vi "STORE_LINEBACK.vi"(9 "CURRENT_YEAR_DATA":string, 10 "ECODE 2":string, 11 "connection reference":T1) -> ()   [LabVIEW 2015]
uses:
  <vilib>/addons/database/Connection.llb/Conn ObjectReference.ctl
  Controls/ITEM_INFORMATION_CLUSTER.ctl
  Controls/Print_Data.ctl
  <vilib>/Instr/_visa.llb/VISA Configure Serial Port (Instr).vi
  <vilib>/addons/database/_DB Variant To Data/Database Variant To Data.xnode
  <vilib>/addons/database/NI_Database_API.lvlib
  <vilib>/addons/database/Connection.llb/DB Tools Open Connec (String).vi
panel:
  in  "Print Button":bool
  in  "BUTTON_ADD":bool
  in  "AUTO PRINT":bool
  in  "Lot Maker":string
  out "Invoice Date":timestamp format="%<%d/%m/%Y>T"
  in  "Location":string
  in  "Scale":refnum<visa-resource-name>
  in  "Tare (g)":dbl
  in  "Weight":dbl
  in  "Sample":dbl caption="Sample (Unit/g)"
  in  "Maker Code":string
  in  "Invoice No.":string
  in  "BUTTON_EXIT":bool
  in  "BUTTON_INPUT":bool
  in  "Unit 2":string
  in  "Quantity":dbl
  in  "Item Code":string
  in  "QR Code (F3)":string
  in  "Maker":string
  in  "Part Name":string
  in  "Product":string
  out "ECODE":string
  out "Lineback Date":timestamp format="%<%d/%m/%Y>T"
  in  "Line No.(F1)":string
  # "INPUT  FROM LINE"
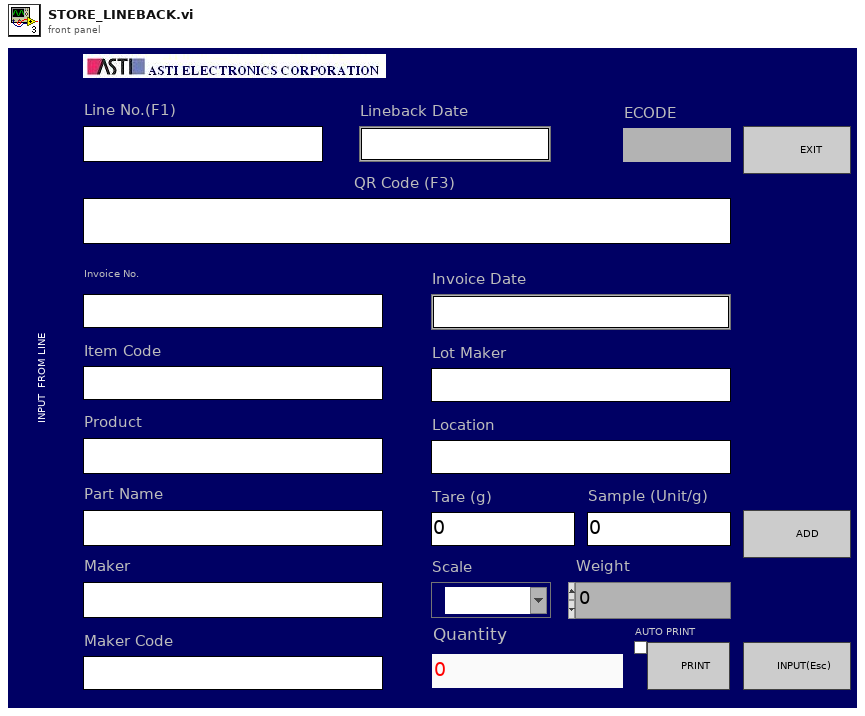
[diagram p1: front panel]
types:
  T1 = typedef "NI_Database_API.lvlib/Conn ObjectReference.ctl" = refnum<k1>
  T2 = cluster{"INVOICE_DATE":timestamp, "LOT_MAKER":string, "INVOICE_NO":string}[]
  T3 = typedef "ITEM_INFORMATION_CLUSTER.ctl" = cluster{"PRODUCT":string, "ITEM_CODE":string, "PART_NAME":string, "MAKER":string, "PART_NO":string, "LOT_SIZE":dbl, "UNIT":string, "LENGTH-OFFSET":string, "BARCODE":string, "PROCESS":string, "INVENTORY_LOCAL":string, "TARE":dbl, "SAMPLE":dbl}
  T4 = cluster{"PRODUCT":string, "ITEM CODE":string, "PART NAME":string, "MAKER":string, "PART NO":string, "LOT SIZE":dbl, "UNIT":string, "LENGTH-OFFSET":string, "BARCODE":string, "PROCESS":string, "INVENTORY LOCAL":string, "TARE":dbl, "SAMPLE":dbl}
  T5 = cluster{"ITEM_CODE":string, "INVOICE_NO":string, "INVOICE_DATE":timestamp, "LOT_MAKER":string, "QUANTITY":dbl, "INVOICE_ECODE":string, "INPUT_NO":string, "INPUT_DATE":timestamp, "INPUT_ECODE":string, "LINEBACK_NO":string, "LINEBACK_DATE":timestamp, "LINEBACK_ECODE":string, "OUTPUT_NO":string, "OUTPUT_DATE":timestamp, "OUTPUT_ECODE":string, "DESTINATION":string}
  T6 = typedef "Print_Data.ctl" = cluster{"QR_code Text":string, "Lot Maker":string, "Item Code (F3)":string, "date/time string":string, "Invoice No.":string, "Maker":string, "Part No.(F2) ":string, "Location":string, "Product":string, "Qty":string, "ECODE":string}
  T7 = cluster{"INVOICE_DATE":timestamp, "LOT_MAKER":string, "INVOICE_NO":string}
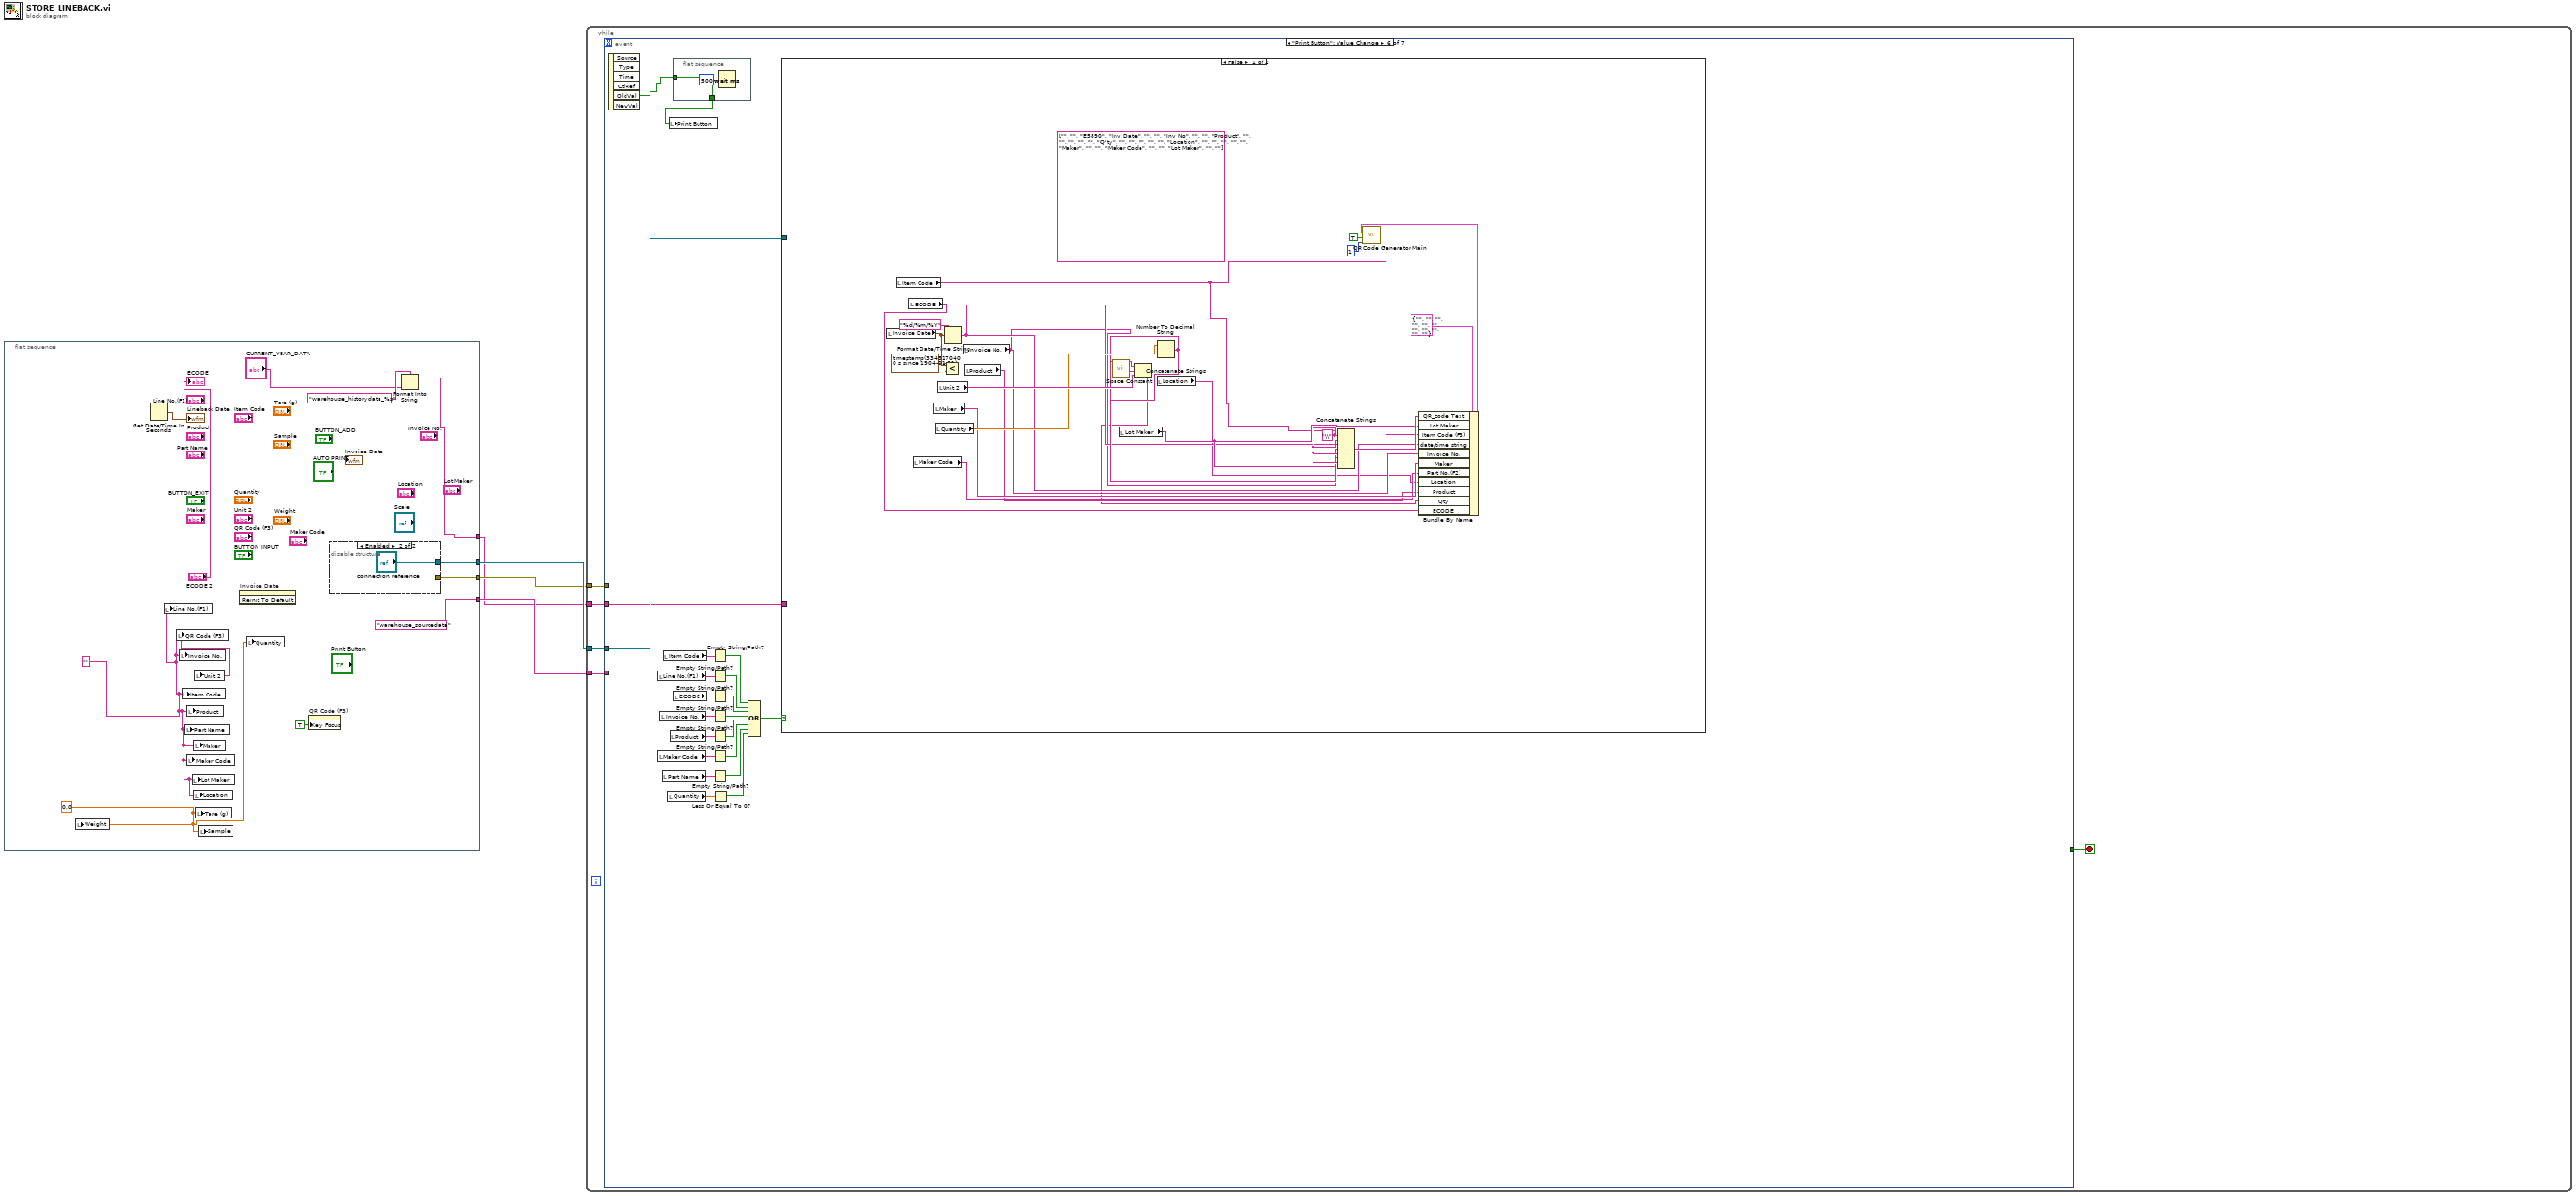
[diagram p0: block diagram]
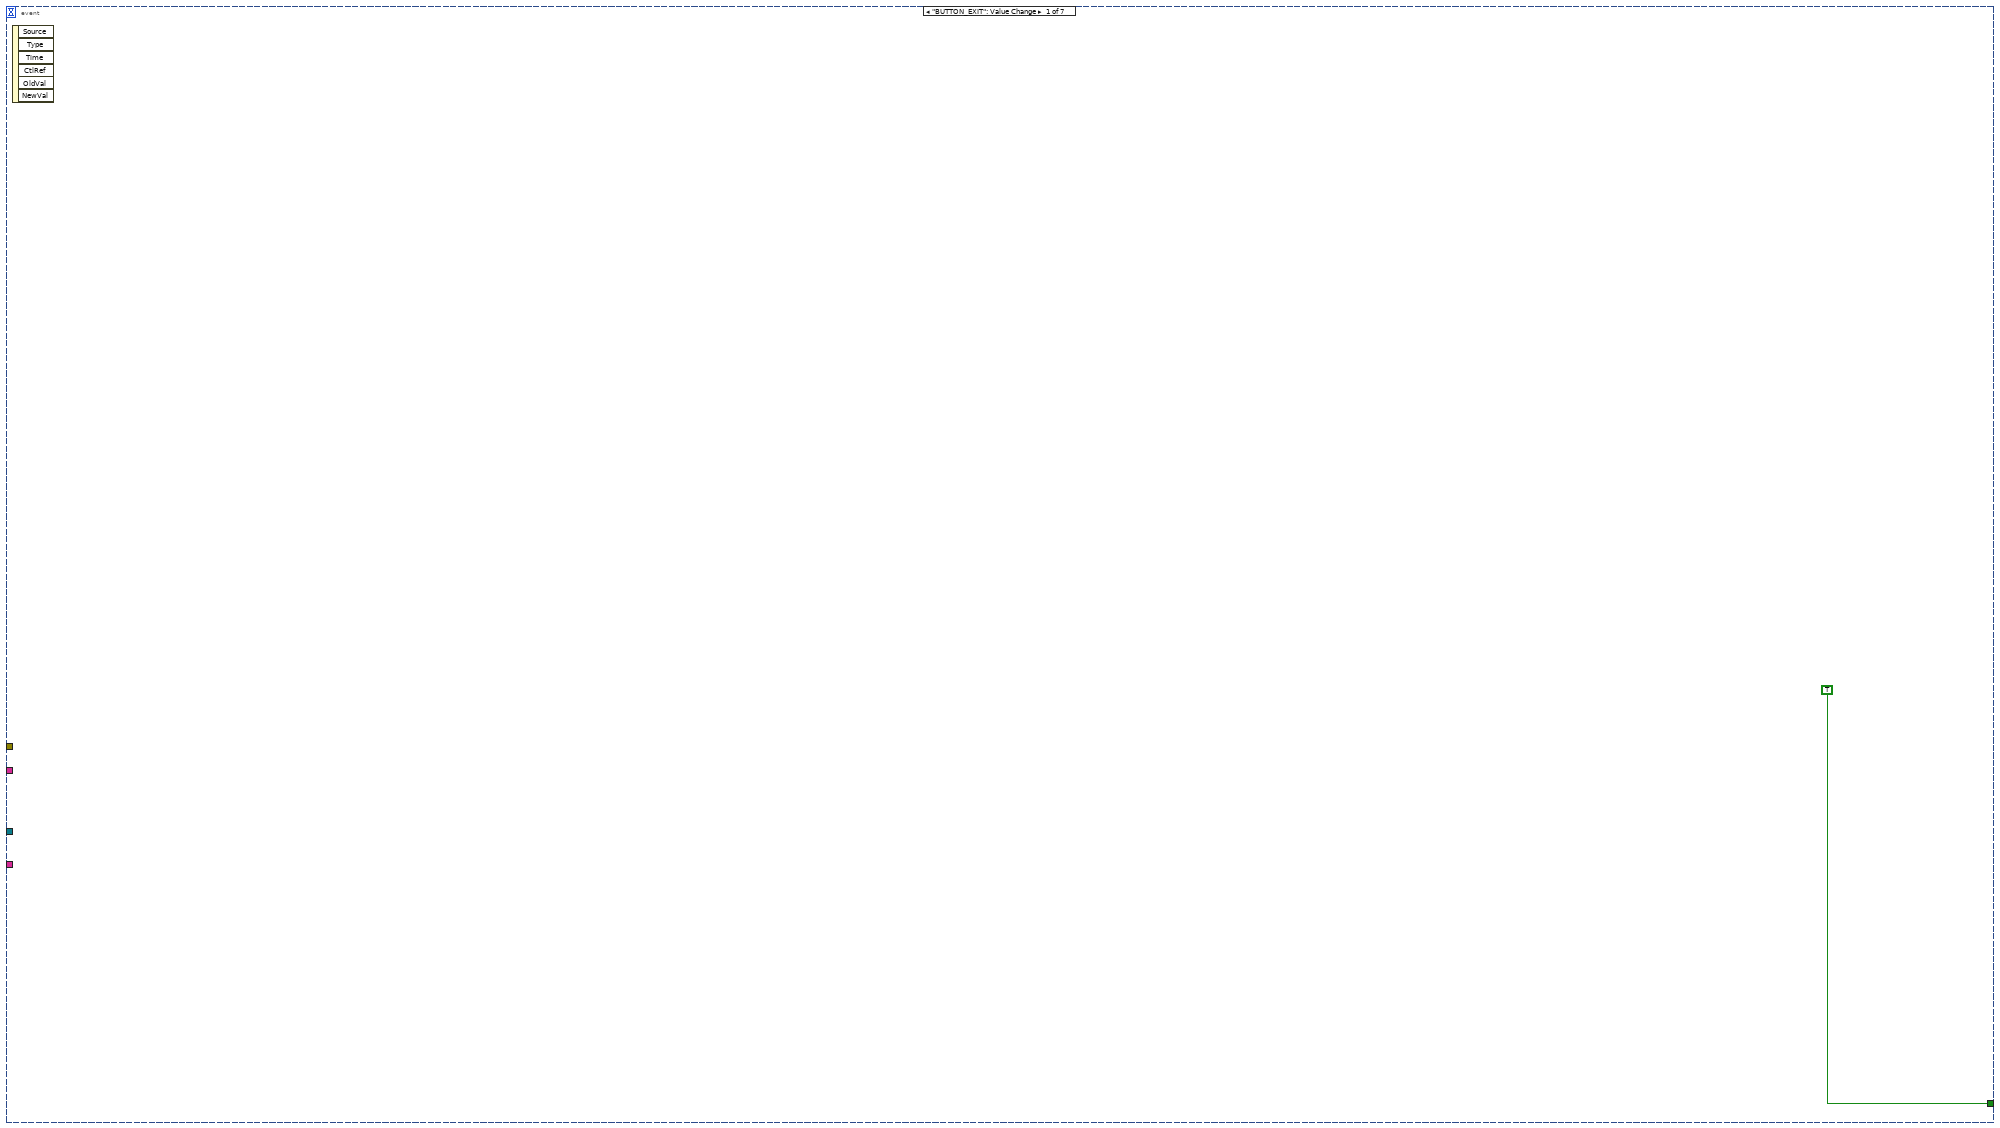
[diagram p2: hidden frame]
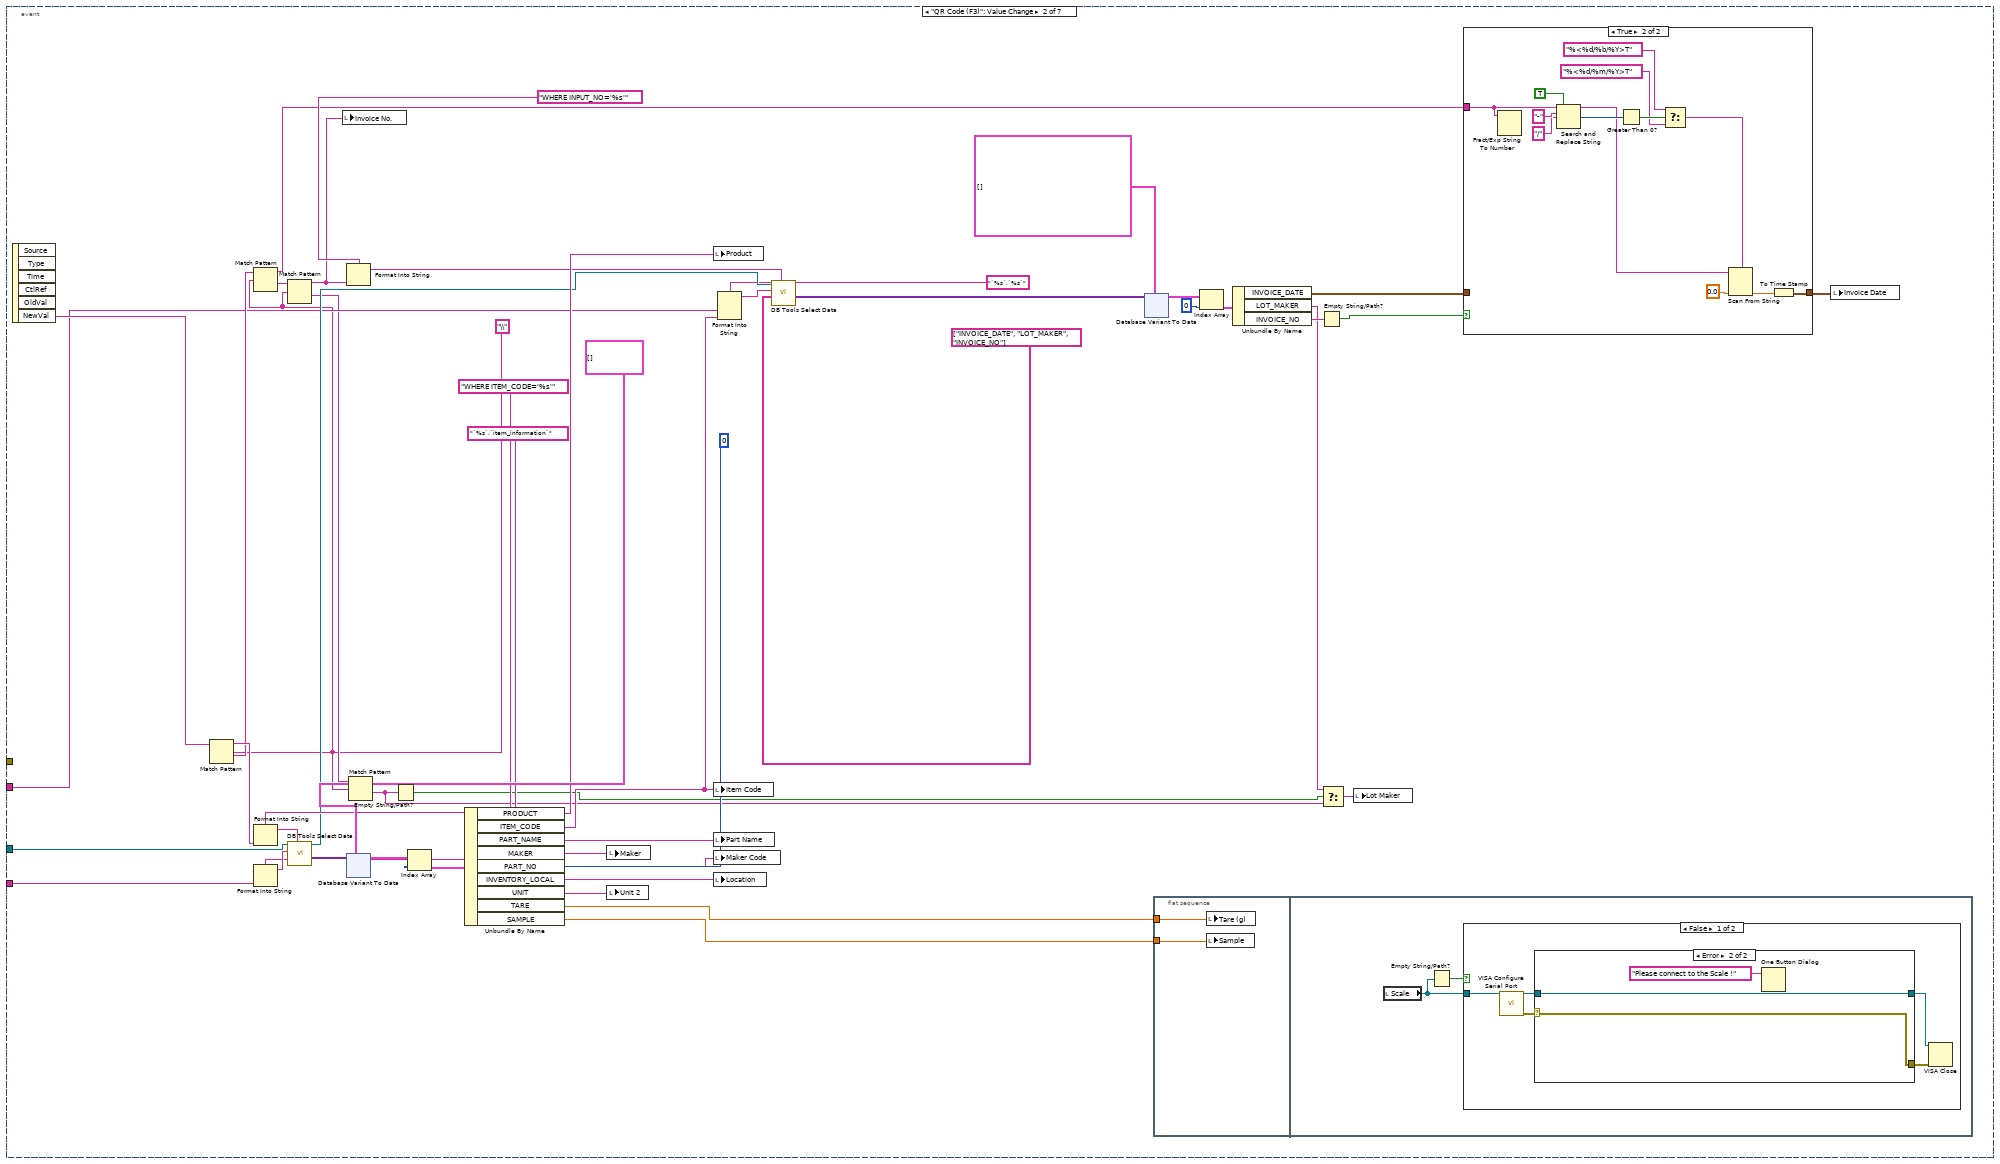
[diagram p3: hidden frame]
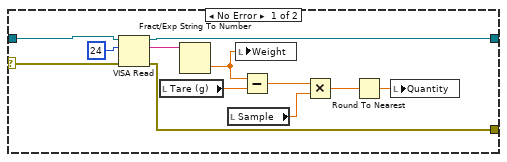
[diagram p5: hidden frame]
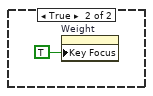
[diagram p6: hidden frame]
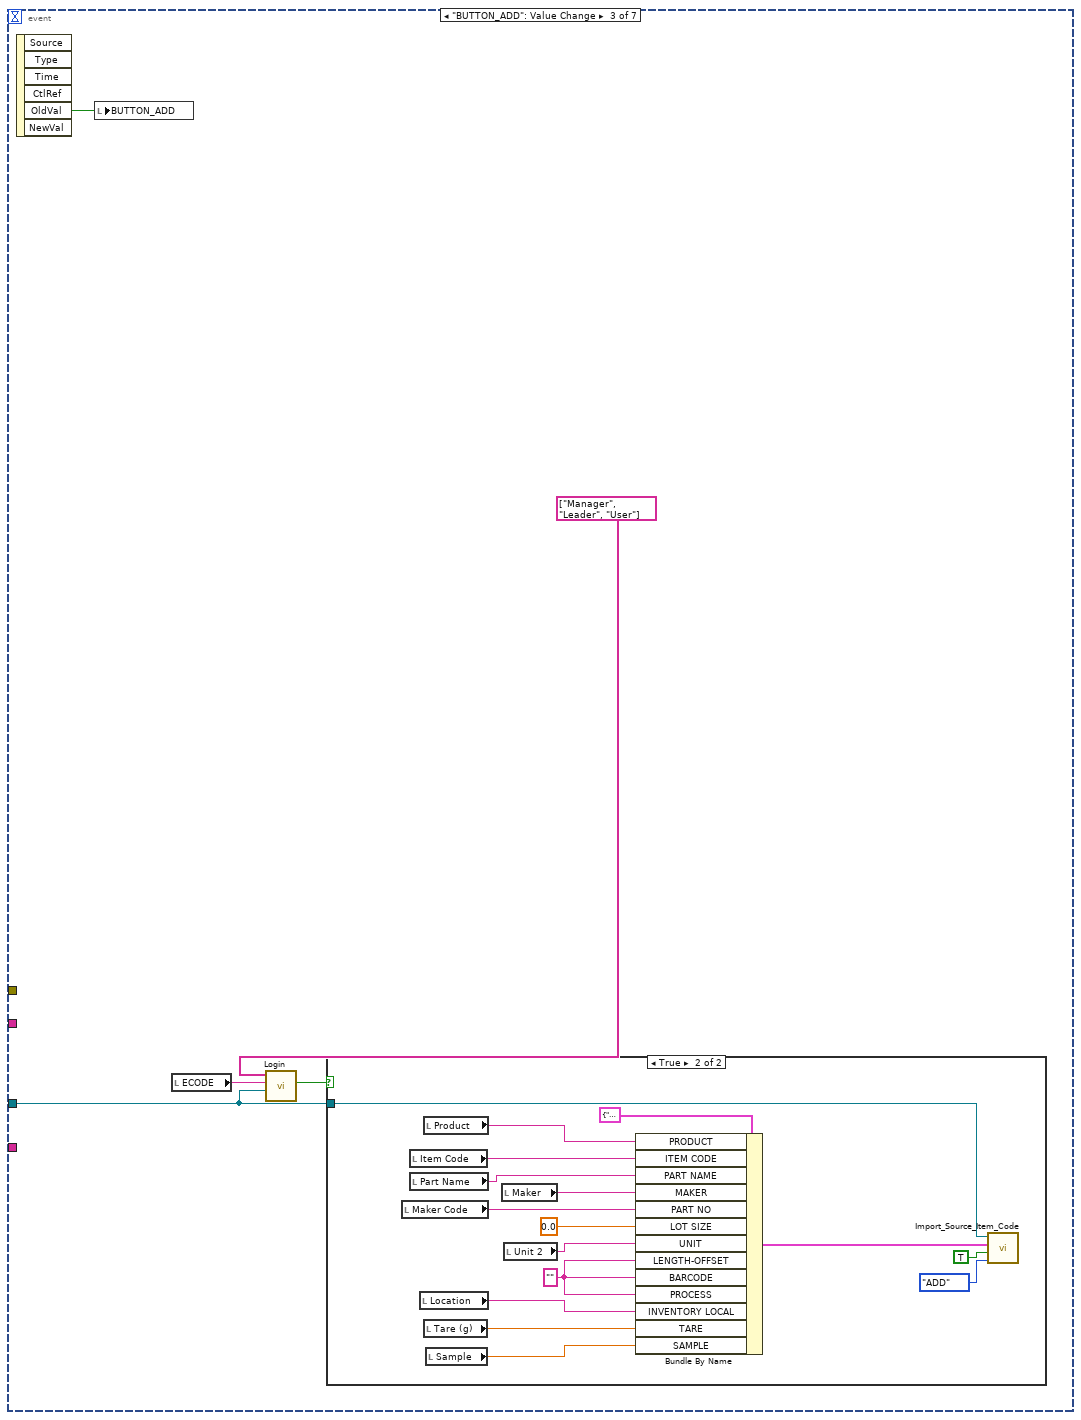
[diagram p7: hidden frame]
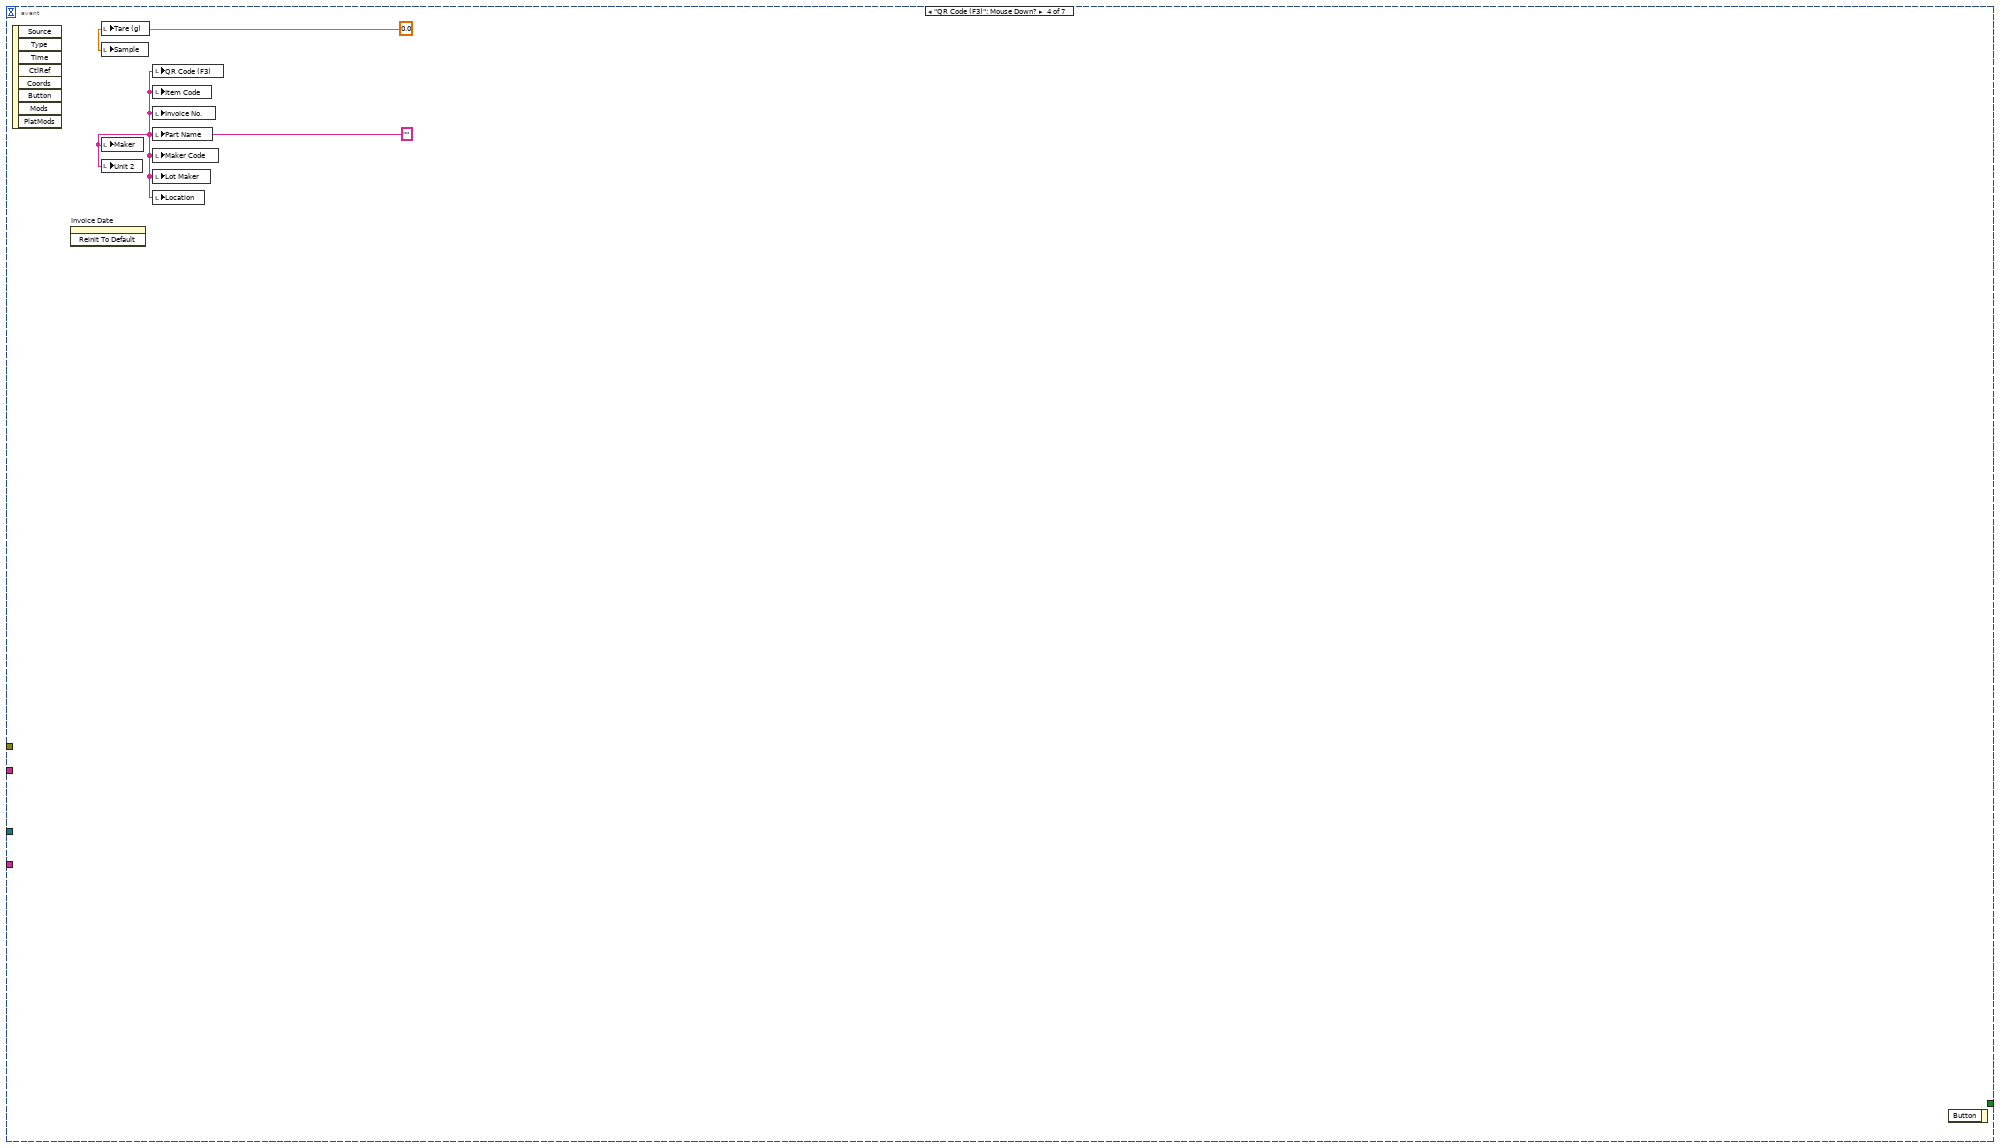
[diagram p9: hidden frame]
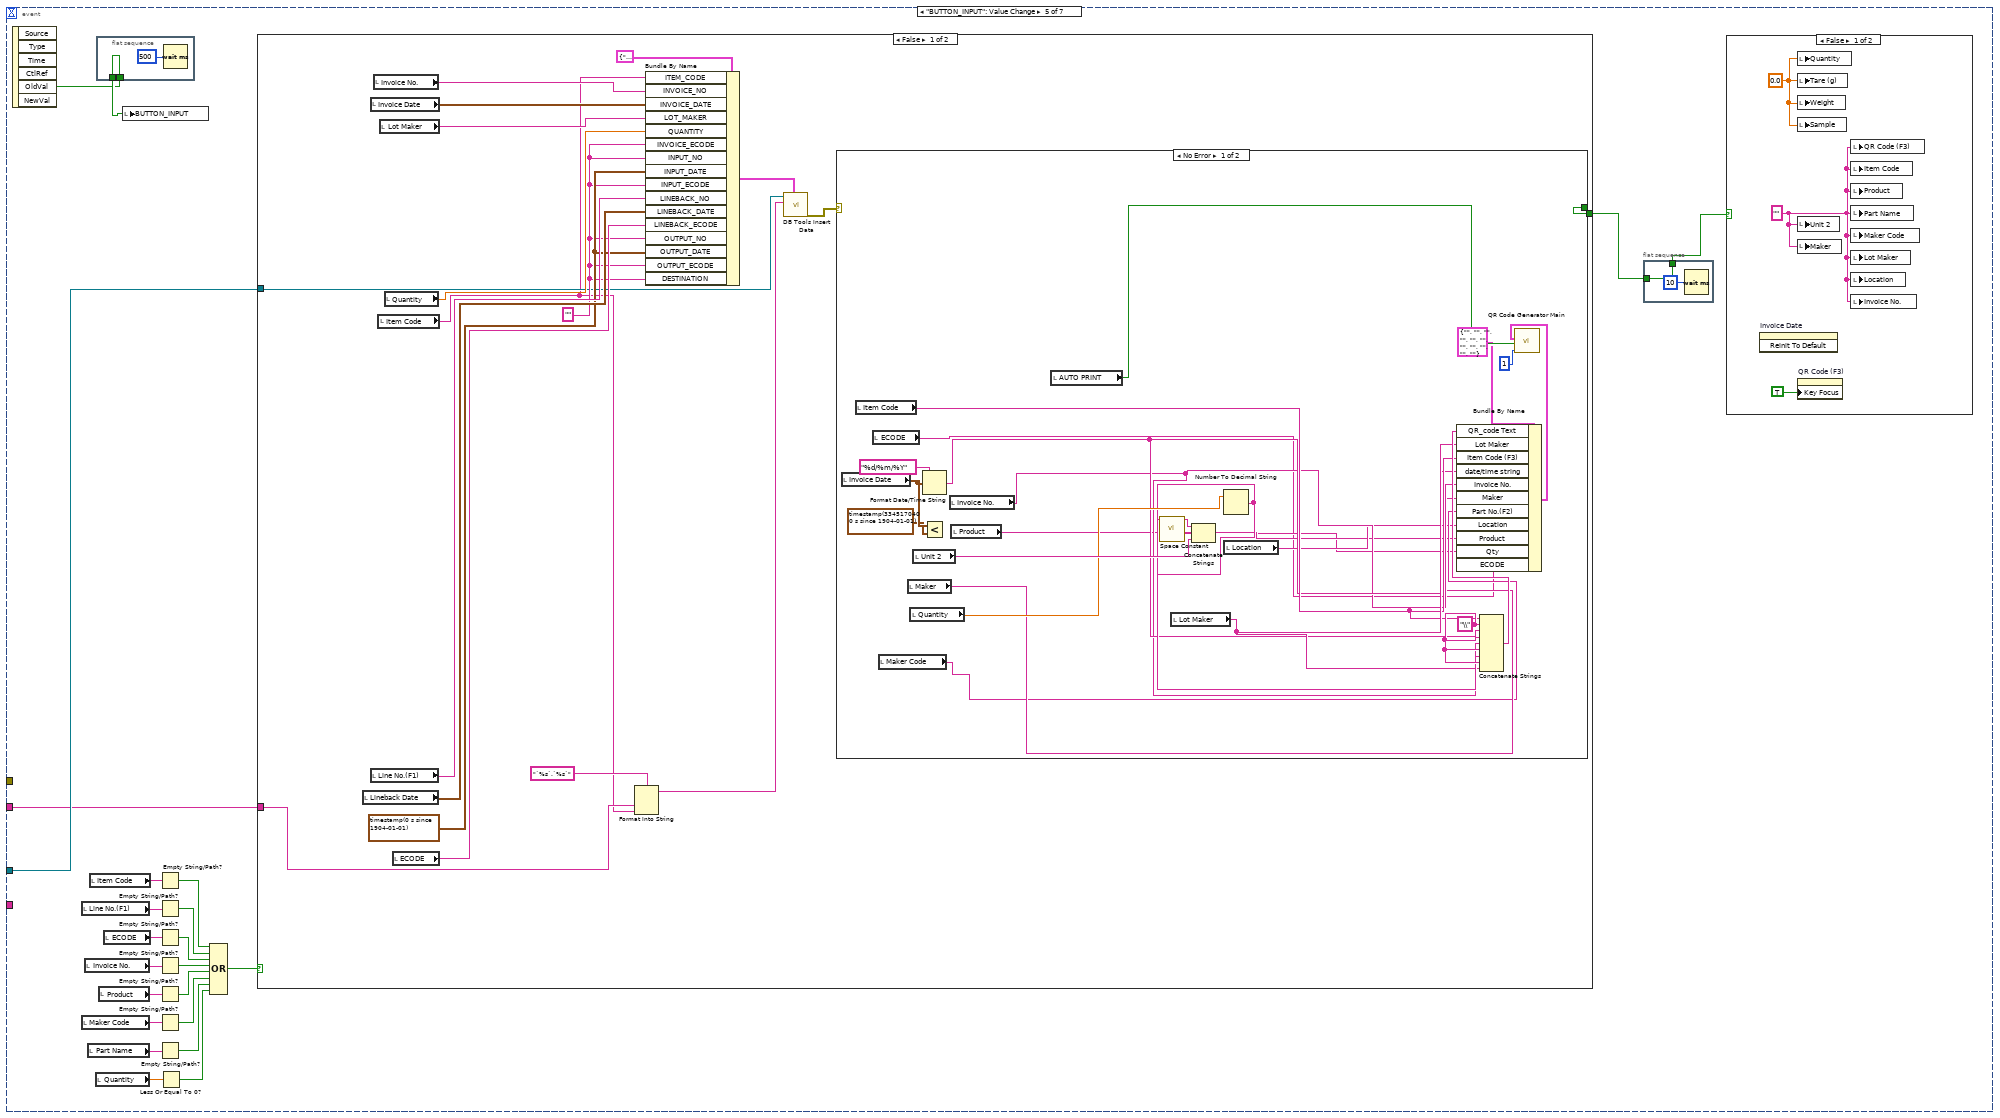
[diagram p10: hidden frame]
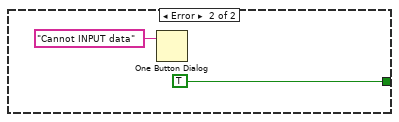
[diagram p12: hidden frame]
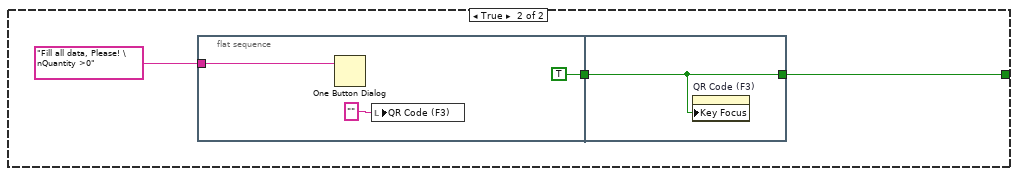
[diagram p13: hidden frame]
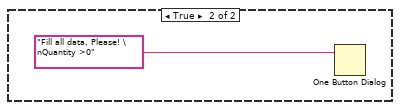
[diagram p14: hidden frame]
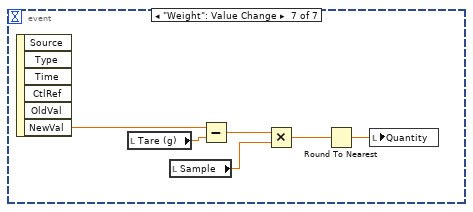
[diagram p15: hidden frame]
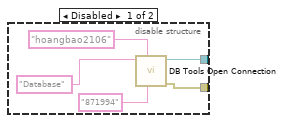
[diagram p16: hidden frame]
diagram:
  n1 = flat-sequence {
    tunnel: [w13] -> w1
    tunnel: [w12] -> w4
    tunnel: [w11] -> w3
    tunnel: ["warehouse_sourcedata" ("table")] -> w2
    frame #0 {
      w6 = ""
      w7 = 0.0
      n2 = local write "Weight"(w7) -> ()
      n3 = Get Date/Time In Seconds() -> (seconds since 1Jan1904=→"Lineback Date":timestamp)
      n4 = local write "Line No.(F1)"(w6) -> ()
      n5 = local write "QR Code (F3)"(w6) -> ()
      n6 = local write "Invoice No."(w6) -> ()
      n7 = local write "Item Code"(w6) -> ()
      n8 = local write "Part Name"(w6) -> ()
      n9 = local write "Maker Code"(w6) -> ()
      n10 = local write "Product"(w6) -> ()
      n11 = local write "Lot Maker"(w6) -> ()
      n12 = local write "Maker"(w6) -> ()
      n13 = local write "Location"(w6) -> ()
      n14 = local write "Unit 2"(w6) -> ()
      n15 = local write "Tare (g)"(w7) -> ()
      n16 = local write "Sample"(w7) -> ()
      n17 = invoke on="Invoice Date" class="AbsTime (strict)" method="Reinit To Default"() -> ()  [unwired: 3 in, 3 out]
      n18 = local write "Quantity"(w7) -> ()
      n19 = property on="QR Code (F3)" class="Str"("Key Focus"=TRUE) -> ()  [unwired: 2 in, 2 out]
      n20 = disable-structure shown="Enabled" {
        disable-tunnel: [w17 "connection reference"] -> w12
        disable-tunnel: [w16 _] -> w11
        frame Disabled {
          n21 = call-poly <vilib>:"DB Tools Open Connection.vi"("password"="871994" ("userID"), "userID"="hoangbao2106", "connection information"="Database" ("userID")) -> ("error out"=w16:errorcluster, "connection reference"=w17:T1)  [unwired: 5 in]
        }
        frame Enabled {
        }
      }
      n22 = Format Into String(format string="warehouse_historydata_%s" ("table"), "CURRENT_YEAR_DATA") -> (resulting string=w13:string)  [unwired: 2 in, 1 out]
      "ECODE" <- "ECODE 2"
    }
  }
  n23 = while {
    tunnel: w4 -> [w25]
    tunnel: w3 -> [w24]
    tunnel: w2 -> [w23]
    tunnel: w1 -> [w22]
    stop <- w26 stop-if-true
    n24 = event shown="[5] \"Print Button\": Value Change" {
      selector: _ -> [_ _ _ _ _ _ _]
      dyn-events: _ -> [_ _ _ _ _ _ _]
      timeout: _ -> [_ _ _ _ _ _ _]
      tunnel: [TRUE _ _ _ _ _ _] -> w26
      tunnel: w25 -> [_ w62 w644 _ w672 w750 _]
      tunnel: w24 -> [_ _ _ _ _ _ _]
      tunnel: w23 -> [_ w61 _ _ _ _ _]
      tunnel: w22 -> [_ w52 _ _ w671 w749 _]
      event "BUTTON_EXIT": Value Change {
        n25 = event-data() -> ()  [unwired: 1 in, 6 out]
      }
      event "QR Code (F3)": Value Change {
        w32 = "\\" ("regular expression")
        n26 = event-data() -> ("NewVal"=w63:string)  [unwired: 1 in, 5 out]
        n27 = Match Pattern(string=w63, regular expression=w32) -> (before substring=w69:string, after substring=w64:string)  [unwired: 1 in, 2 out]
        n28 = Match Pattern(string=w64, regular expression=w32) -> (before substring=w36:string, after substring=w65:string)  [unwired: 1 in, 2 out]
        n29 = Format Into String(format string="WHERE ITEM_CODE='%s'", w69) -> (resulting string=w70:string)  [unwired: 2 in, 1 out]
        n30 = Format Into String(format string="`%s`.`item_information`", w61) -> (resulting string=w67:string)  [unwired: 2 in, 1 out]
        n31 = Match Pattern(string=w65, regular expression=w32) -> (before substring=w48:string, after substring=w33:string)  [unwired: 1 in, 2 out]
        n32 = call <vilib>:"DB Tools Select Data.vi"("condition"=w70, "table"=w67, "connection reference"=w62) -> ("data"=w71:variant[][], "connection reference out"=w54:T1)  [unwired: 3 in, 1 out]
        n33 = local write "Invoice No."(w48) -> ()
        n34 = xnode "Database Variant To Data"("database variant"=w71, "type"=T3[] []) -> ("data"=w73:T3[])  [unwired: 1 in, 1 out]
        n35 = Format Into String(format string="WHERE INPUT_NO='%s'", w48) -> (resulting string=w49:string)  [unwired: 2 in, 1 out]
        n36 = Match Pattern(string=w33, regular expression=w32) -> (after substring=w28:string)  [unwired: 1 in, 3 out]
        n37 = Empty String/Path?(string/path=w28) -> (empty?=w31:bool)
        n38 = Index Array(array=w73, index=0) -> (element=w75:T3)
        n39 = Unbundle By Name(w75) -> ("PRODUCT"=w60:string, "ITEM_CODE"=w47:string, "PART_NAME"=w59:string, "MAKER"=w57:string, "PART_NO"=w58:string, "INVENTORY_LOCAL"=w56:string, "UNIT"=w55:string, "TARE"=w41:dbl, "SAMPLE"=w40:dbl)
        n40 = local write "Maker"(w57) -> ()
        n41 = local write "Unit 2"(w55) -> ()
        n42 = local write "Product"(w60) -> ()
        n43 = local write "Item Code"(w47) -> ()
        n44 = local write "Part Name"(w59) -> ()
        n45 = local write "Maker Code"(w58) -> ()
        n46 = local write "Location"(w56) -> ()
        n47 = Format Into String(format string="`%s`.`%s`", w52, w47) -> (resulting string=w51:string)  [unwired: 2 in, 1 out]
        n48 = call <vilib>:"DB Tools Select Data.vi"("condition"=w49, "columns"=string[] ["INVOICE_DATE", "LOT_MAKER", "INVOICE_NO"], "table"=w51, "connection reference"=w54) -> ("data"=w46:variant[][])  [unwired: 2 in, 2 out]
        n49 = xnode "Database Variant To Data"("database variant"=w46, "type"=T2 []) -> ("data"=w43:T2)  [unwired: 1 in, 1 out]
        n50 = flat-sequence {
          tunnel: w41 -> [w91]
          tunnel: w40 -> [w90]
          frame #0 {
            n51 = local write "Tare (g)"(w91) -> ()
            n52 = local write "Sample"(w90) -> ()
          }
          frame #1 {
            n53 = local read "Scale"() -> (w92:refnum<visa-resource-name>)
            n54 = Empty String/Path?(string/path=w92) -> (empty?=w93:bool)
            n55 = case shown="False" w93 {
              tunnel: w92 -> [w94 _]
              frame False {
                n56 = call-poly "VISA Configure Serial Port"("VISA resource name"=w94) -> ("VISA resource name out"=w97:refnum<visa-resource-name>, "error out"=w98:errorcluster)  [unwired: 13 in]
                n57 = case shown="Error" w98 {
                  selector: w98 -> [w109 w112]
                  tunnel: w97 -> [w110 w113]
                  tunnel: [w108 w113] -> w96
                  tunnel: [w107 w112] -> w95
                  frame No Error {
                    n58 = VISA Read(VISA resource name=w110, byte count=u32 24, error in (no error)=w109) -> (VISA resource name out=w108:refnum<visa-resource-name>, read buffer=w105:string, error out=w107:errorcluster)  [unwired: 1 out]
                    n59 = local read "Tare (g)"() -> (w101:dbl)
                    n60 = Fract/Exp String To Number(string=w105) -> (number=w99:dbl)  [unwired: 3 in, 1 out]
                    n61 = local read "Sample"() -> (w102:dbl)
                    n62 = local write "Weight"(w99) -> ()
                    n63 = Subtract(x=w99, y=w101) -> (x-y=w103:dbl)
                    n64 = Multiply(x=w103, y=w102) -> (x*y=w104:dbl)
                    n65 = Round To Nearest(number=w104) -> (nearest integer value=w100:dbl)
                    n66 = local write "Quantity"(w100) -> ()
                  }
                  frame Error {
                    n67 = One Button Dialog(message="Please connect to the Scale !") -> ()  [unwired: 1 in, 1 out]
                  }
                }
                n68 = VISA Close(VISA resource name=w96, error in (no error)=w95) -> ()  [unwired: 1 out]
              }
              frame True {
                n69 = property on="Weight" class="DigNum (strict)"("Key Focus"=TRUE) -> ()  [unwired: 2 in, 2 out]
              }
            }
          }
        }
        n70 = Index Array(array=w43, index=0 ("index (row)")) -> (element=w39:T7)
        n71 = Unbundle By Name(w39) -> ("INVOICE_DATE"=w34:timestamp, "LOT_MAKER"=w29:string, "INVOICE_NO"=w38:string)
        n72 = Empty String/Path?(string/path=w38) -> (empty?=w37:bool)
        n73 = Select(t=w29, s=w31, f=w28) -> (s? t:f=w30:string)
        n74 = local write "Lot Maker"(w30) -> ()
        n75 = case shown="True" w37 {
          tunnel: w36 -> [_ w88]
          tunnel: [w76 w89] -> w35
          tunnel: w34 -> [w76 _]
          frame False {
          }
          frame True {
            n76 = Fract/Exp String To Number(string=w88) -> ()  [unwired: 3 in, 2 out]
            n77 = Search and Replace String(replace all?=TRUE ("replace all? (F)"), input string=w88, search string="-", replace string="/" ("replace string (\"\")")) -> (result string=w77:string, number of replacements=w84:i32)  [unwired: 4 in, 2 out]
            n78 = Greater Than 0?(x=w84) -> (x > 0?=w83:bool)
            n79 = Select(t="%<%d/%b/%Y>T" ("format string"), s=w83, f="%<%d/%m/%Y>T" ("format string")) -> (s? t:f=w78:string)
            n80 = Scan From String(format string=w78, input string=w77, default 1=0.0) -> (output 1=w80:dbl)  [unwired: 2 in, 3 out]
            n81 = To Time Stamp(1:w80) -> (0:w89:timestamp)
          }
        }
        n82 = local write "Invoice Date"(w35) -> ()
      }
      event "BUTTON_ADD": Value Change {
        n83 = event-data() -> ("OldVal"=w648:bool)  [unwired: 1 in, 5 out]
        n84 = local write "BUTTON_ADD"(w648) -> ()
        n85 = local read "ECODE"() -> (w647:string)
        n86 = call "Login.vi"("connection reference"=w644, "ACCOUNT:"=w647, "Permission"=string[] ["Manager", "Leader", "User"]) -> ("OK"=w646:bool)  [unwired: 7 in, 1 out]
        n87 = case shown="True" w646 {
          tunnel: w644 -> [_ w664]
          frame False {
          }
          frame True {
            w651 = "" ("PROCESS")
            n88 = local read "Maker Code"() -> (w658:string)
            n89 = local read "Item Code"() -> (w661:string)
            n90 = local read "Part Name"() -> (w660:string)
            n91 = local read "Location"() -> (w656:string)
            n92 = local read "Product"() -> (w662:string)
            n93 = local read "Tare (g)"() -> (w650:dbl)
            n94 = local read "Sample"() -> (w649:dbl)
            n95 = local read "Maker"() -> (w659:string)
            n96 = local read "Unit 2"() -> (w657:string)
            n97 = Bundle By Name(cluster=T4 {"PRODUCT"="", "ITEM CODE"="", "PART NAME"="", "MAKER"="", "PART NO"="", "LOT SIZE"=0.0, "UNIT"="", "LENGTH-OFFSET"="", "BARCODE"="", "PROCESS"="", "INVENTORY LOCAL"="", "TARE"=0.0, "SAMPLE"=0.0} ("ITEM_DATA"), "PRODUCT"=w662, "ITEM CODE"=w661, "PART NAME"=w660, "MAKER"=w659, "PART NO"=w658, "LOT SIZE"=0.0 ("TARE"), "UNIT"=w657, "LENGTH-OFFSET"=w651, "BARCODE"=w651, "PROCESS"=w651, "INVENTORY LOCAL"=w656, "TARE"=w650, "SAMPLE"=w649) -> (w653:T4)
            n98 = call "Import_Source_Item_Code.vi"("CONTROL Control"=enum32{"IMPRORT", "ADD"}."ADD", "UPDATE ONLY"=TRUE, "ITEM_DATA"=w653, "connection reference"=w664) -> ()  [unwired: 8 in]
          }
        }
      }
      event "QR Code (F3)": Mouse Down? {
        w666 = 0.0
        w665 = ""
        n99 = event-data() -> ()  [unwired: 1 in, 8 out]
        n100 = invoke on="Invoice Date" class="AbsTime (strict)" method="Reinit To Default"() -> ()  [unwired: 3 in, 3 out]
        n101 = local write "Tare (g)"(w666) -> ()
        n102 = local write "Sample"(w666) -> ()
        n103 = local write "Maker"(w665) -> ()
        n104 = local write "Unit 2"(w665) -> ()
        n105 = local write "QR Code (F3)"(w665) -> ()
        n106 = local write "Item Code"(w665) -> ()
        n107 = local write "Invoice No."(w665) -> ()
        n108 = local write "Part Name"(w665) -> ()
        n109 = local write "Maker Code"(w665) -> ()
        n110 = local write "Lot Maker"(w665) -> ()
        n111 = local write "Location"(w665) -> ()
        n112 = event-data() -> ()  [unwired: 2 in, 1 out]
      }
      event "BUTTON_INPUT": Value Change {
        n113 = event-data() -> ("OldVal"=w667:bool)  [unwired: 1 in, 5 out]
        n114 = local read "Line No.(F1)"() -> (w689:string)
        n115 = local read "Maker Code"() -> (w685:string)
        n116 = local read "Invoice No."() -> (w687:string)
        n117 = local read "Part Name"() -> (w684:string)
        n118 = local read "Item Code"() -> (w674:string)
        n119 = local read "Quantity"() -> (w683:dbl)
        n120 = flat-sequence {
          tunnel: [w691] -> w668
          tunnel: w667 -> [w691]
          frame #0 {
            n121 = Wait (ms)(milliseconds to wait=u32 500) -> ()  [unwired: 1 out]
          }
        }
        n122 = local read "Product"() -> (w686:string)
        n123 = local read "ECODE"() -> (w688:string)
        n124 = local write "BUTTON_INPUT"(w668) -> ()
        n125 = Empty String/Path?(string/path=w674) -> (empty?=w673:bool)
        n126 = Empty String/Path?(string/path=w689) -> (empty?=w682:bool)
        n127 = Empty String/Path?(string/path=w688) -> (empty?=w681:bool)
        n128 = Empty String/Path?(string/path=w687) -> (empty?=w680:bool)
        n129 = Empty String/Path?(string/path=w686) -> (empty?=w679:bool)
        n130 = Empty String/Path?(string/path=w685) -> (empty?=w678:bool)
        n131 = Empty String/Path?(string/path=w684) -> (empty?=w677:bool)
        n132 = Less Or Equal To 0?(x=w683) -> (x <= 0?=w676:bool)
        n133 = Compound Arithmetic op=OR(w673, w682, w681, w680, w679, w678, w677, w676) -> (w675:bool)
        n134 = case shown="False" w675 {
          tunnel: w672 -> [w704 _]
          tunnel: w671 -> [w702 _]
          tunnel: [w697 w740] -> w670
          frame False {
            w705 = ""
            w706 = timestamp(0 s since 1904-01-01)
            n135 = local read "Lineback Date"() -> (w708:timestamp)
            n136 = local read "Invoice Date"() -> (w712:timestamp)
            n137 = local read "Line No.(F1)"() -> (w709:string)
            n138 = local read "Invoice No."() -> (w713:string)
            n139 = local read "Item Code"() -> (w701:string)
            n140 = local read "Lot Maker"() -> (w711:string)
            n141 = local read "Quantity"() -> (w710:dbl)
            n142 = local read "ECODE"() -> (w707:string)
            n143 = Format Into String(format string="`%s`.`%s`", w702, w701) -> (resulting string=w700:string)  [unwired: 2 in, 1 out]
            n144 = Bundle By Name(cluster=T5 {"ITEM_CODE"="", "INVOICE_NO"="", "INVOICE_DATE"=timestamp(0 s since 1904-01-01), "LOT_MAKER"="", "QUANTITY"=0.0, "INVOICE_ECODE"="", "INPUT_NO"="", "INPUT_DATE"=timestamp(0 s since 1904-01-01), "INPUT_ECODE"="", "LINEBACK_NO"="", "LINEBACK_DATE"=timestamp(0 s since 1904-01-01), "LINEBACK_ECODE"="", "OUTPUT_NO"="", "OUTPUT_DATE"=timestamp(0 s since 1904-01-01), "OUTPUT_ECODE"="", "DESTINATION"=""}, "ITEM_CODE"=w701, "INVOICE_NO"=w713, "INVOICE_DATE"=w712, "LOT_MAKER"=w711, "QUANTITY"=w710, "INVOICE_ECODE"=w705, "INPUT_NO"=w705, "INPUT_DATE"=w706, "INPUT_ECODE"=w705, "LINEBACK_NO"=w709, "LINEBACK_DATE"=w708, "LINEBACK_ECODE"=w707, "OUTPUT_NO"=w705, "OUTPUT_DATE"=w706, "OUTPUT_ECODE"=w705, "DESTINATION"=w705) -> (w699:T5)
            n145 = call <vilib>:"DB Tools Insert Data.vi"("data"=w699, "table"=w700, "connection reference"=w704) -> ("error out"=w698:errorcluster)  [unwired: 7 in, 1 out]
            n146 = case shown="No Error" w698 {
              tunnel: [_ TRUE] -> w697
              frame No Error {
                w732 = "\\" ("string")
                n147 = local read "Invoice Date"() -> (w736:timestamp)
                n148 = local read "Item Code"() -> (w724:string)
                n149 = local read "ECODE"() -> (w716:string)
                n150 = local read "Maker Code"() -> (w720:string)
                n151 = local read "Maker"() -> (w721:string)
                n152 = local read "Quantity"() -> (w733:dbl)
                n153 = local read "Unit 2"() -> (w734:string)
                n154 = Format Date/Time String(time format string (%c)="%d/%m/%Y", seconds (now)=w736) -> (date/time string=w723:string)  [unwired: 1 in]
                n155 = Less?(x=w736, y=timestamp(3345170400 s since 1904-01-01)) -> ()  [unwired: 1 out]
                n156 = local read "Invoice No."() -> (w722:string)
                n157 = local read "Product"() -> (w718:string)
                n158 = local read "AUTO PRINT"() -> (w728:bool)
                n159 = call <vilib>:"Space Constant.vi"() -> ("String"=w731:string)
                n160 = local read "Lot Maker"() -> (w725:string)
                n161 = Number To Decimal String(number=w733) -> (decimal integer string=w730:string)  [unwired: 1 in]
                n162 = Concatenate Strings(w730, w731, w734) -> (w717:string)
                n163 = local read "Location"() -> (w719:string)
                n164 = Concatenate Strings(w724, w732, w723, w732, w722, w732, w730, w732, w725) -> (w726:string)
                n165 = Bundle By Name(cluster=T6 {"QR_code Text"="", "Lot Maker"="", "Item Code (F3)"="", "date/time string"="", "Invoice No."="", "Maker"="", "Part No.(F2) "="", "Location"="", "Product"="", "Qty"="", "ECODE"=""} ("output cluster"), "QR_code Text"=w726, "Lot Maker"=w725, "Item Code (F3)"=w724, "date/time string"=w723, "Invoice No."=w722, "Maker"=w721, "Part No.(F2)"=w720, "Location"=w719, "Product"=w718, "Qty"=w717, "ECODE"=w716) -> (w715:T6)
                n166 = call "QR Code Generator Main.vi"("number of copies (1)"=1, "Print Button"=w728, "output cluster"=w715) -> ()  [unwired: 9 in]
              }
              frame Error {
                n167 = One Button Dialog(message="Cannot INPUT data") -> ()  [unwired: 1 in, 1 out]
              }
            }
          }
          frame True {
            n168 = flat-sequence {
              tunnel: "Fill all data, Please! \nQuantity >0" ("message") -> [w745]
              tunnel: [TRUE ("Key Focus")] -> w742
              tunnel: w742 -> [w746]
              tunnel: [w746] -> w740
              frame #0 {
                n169 = One Button Dialog(message=w745) -> ()  [unwired: 1 in, 1 out]
                n170 = local write "QR Code (F3)"("" ("QR Code")) -> ()
              }
              frame #1 {
                n171 = property on="QR Code (F3)" class="Str"("Key Focus"=w746) -> ()  [unwired: 2 in, 2 out]
              }
            }
          }
        }
        n172 = flat-sequence {
          tunnel: [w693] -> w669
          tunnel: w670 -> [w693]
          frame #0 {
            n173 = Wait (ms)(milliseconds to wait=u32 10) -> ()  [unwired: 1 out]
          }
        }
        n174 = case shown="False" w669 {
          frame False {
            w696 = ""
            w695 = 0.0
            n175 = invoke on="Invoice Date" class="AbsTime (strict)" method="Reinit To Default"() -> ()  [unwired: 3 in, 3 out]
            n176 = local write "Quantity"(w695) -> ()
            n177 = local write "Tare (g)"(w695) -> ()
            n178 = local write "Weight"(w695) -> ()
            n179 = local write "Sample"(w695) -> ()
            n180 = local write "Unit 2"(w696) -> ()
            n181 = local write "Maker"(w696) -> ()
            n182 = property on="QR Code (F3)" class="Str"("Key Focus"=TRUE) -> ()  [unwired: 2 in, 2 out]
            n183 = local write "QR Code (F3)"(w696) -> ()
            n184 = local write "Item Code"(w696) -> ()
            n185 = local write "Product"(w696) -> ()
            n186 = local write "Part Name"(w696) -> ()
            n187 = local write "Maker Code"(w696) -> ()
            n188 = local write "Lot Maker"(w696) -> ()
            n189 = local write "Location"(w696) -> ()
            n190 = local write "Invoice No."(w696) -> ()
          }
          frame True {
          }
        }
      }
      event "Print Button": Value Change {
        n191 = event-data() -> ("OldVal"=w748:bool)  [unwired: 1 in, 5 out]
        n192 = local read "Line No.(F1)"() -> (w767:string)
        n193 = local read "Maker Code"() -> (w763:string)
        n194 = local read "Invoice No."() -> (w765:string)
        n195 = local read "Part Name"() -> (w762:string)
        n196 = local read "Item Code"() -> (w752:string)
        n197 = local read "Quantity"() -> (w761:dbl)
        n198 = local write "Print Button"(w747) -> ()
        n199 = local read "Product"() -> (w764:string)
        n200 = flat-sequence {
          tunnel: [w769] -> w747
          tunnel: w748 -> [w769]
          frame #0 {
            n201 = Wait (ms)(milliseconds to wait=u32 500) -> ()  [unwired: 1 out]
          }
        }
        n202 = local read "ECODE"() -> (w766:string)
        n203 = Empty String/Path?(string/path=w752) -> (empty?=w751:bool)
        n204 = Empty String/Path?(string/path=w767) -> (empty?=w760:bool)
        n205 = Empty String/Path?(string/path=w766) -> (empty?=w759:bool)
        n206 = Empty String/Path?(string/path=w765) -> (empty?=w758:bool)
        n207 = Empty String/Path?(string/path=w764) -> (empty?=w757:bool)
        n208 = Empty String/Path?(string/path=w763) -> (empty?=w756:bool)
        n209 = Empty String/Path?(string/path=w762) -> (empty?=w755:bool)
        n210 = Less Or Equal To 0?(x=w761) -> (x <= 0?=w754:bool)
        n211 = Compound Arithmetic op=OR(w751, w760, w759, w758, w757, w756, w755, w754) -> (w753:bool)
        n212 = case shown="False" w753 {
          tunnel: w750 -> [_ _]
          tunnel: w749 -> [_ _]
          frame False {
            w787 = "\\" ("string")
            (unwired) string[][] [["", "", "E5890"], ["Inv Date", "", ""], ["Inv No", "", ""], ["Product", "", ""], ["", "", ""], ["Q'ty", "", ""], ["", "", ""], ["Location", "", ""], ["", "", ""], ["Maker", "", ""], ["Maker Code", "", ""], ["Lot Maker", "", ""]] ("Text Label")
            n213 = local read "Invoice Date"() -> (w791:timestamp)
            n214 = local read "Item Code"() -> (w779:string)
            n215 = local read "ECODE"() -> (w771:string)
            n216 = local read "Maker Code"() -> (w775:string)
            n217 = local read "Maker"() -> (w776:string)
            n218 = local read "Quantity"() -> (w788:dbl)
            n219 = local read "Unit 2"() -> (w789:string)
            n220 = Format Date/Time String(time format string (%c)="%d/%m/%Y", seconds (now)=w791) -> (date/time string=w778:string)  [unwired: 1 in]
            n221 = Less?(x=w791, y=timestamp(3345170400 s since 1904-01-01)) -> ()  [unwired: 1 out]
            n222 = local read "Invoice No."() -> (w777:string)
            n223 = local read "Product"() -> (w773:string)
            n224 = call <vilib>:"Space Constant.vi"() -> ("String"=w786:string)
            n225 = local read "Lot Maker"() -> (w780:string)
            n226 = Number To Decimal String(number=w788) -> (decimal integer string=w785:string)  [unwired: 1 in]
            n227 = Concatenate Strings(w785, w786, w789) -> (w772:string)
            n228 = local read "Location"() -> (w774:string)
            n229 = Concatenate Strings(w779, w787, w778, w787, w777, w787, w785, w787, w780) -> (w781:string)
            n230 = Bundle By Name(cluster=T6 {"QR_code Text"="", "Lot Maker"="", "Item Code (F3)"="", "date/time string"="", "Invoice No."="", "Maker"="", "Part No.(F2) "="", "Location"="", "Product"="", "Qty"="", "ECODE"=""} ("output cluster"), "QR_code Text"=w781, "Lot Maker"=w780, "Item Code (F3)"=w779, "date/time string"=w778, "Invoice No."=w777, "Maker"=w776, "Part No.(F2)"=w775, "Location"=w774, "Product"=w773, "Qty"=w772, "ECODE"=w771) -> (w770:T6)
            n231 = call "QR Code Generator Main.vi"("number of copies (1)"=1, "Print Button"=TRUE, "output cluster"=w770) -> ()  [unwired: 9 in]
          }
          frame True {
            n232 = One Button Dialog(message="Fill all data, Please! \nQuantity >0") -> ()  [unwired: 1 in, 1 out]
          }
        }
      }
      event "Weight": Value Change {
        n233 = event-data() -> ("NewVal"=w799:dbl)  [unwired: 1 in, 5 out]
        n234 = local read "Tare (g)"() -> (w798:dbl)
        n235 = local read "Sample"() -> (w796:dbl)
        n236 = Subtract(x=w799, y=w798) -> (x-y=w797:dbl)
        n237 = Multiply(x=w797, y=w796) -> (x*y=w795:dbl)
        n238 = Round To Nearest(number=w795) -> (nearest integer value=w794:dbl)
        n239 = local write "Quantity"(w794) -> ()
      }
    }
  }
